vi "GOOP300_GetClassTemplatePath.vi"(1 "ClassTemplateSubDirectory":string, 5 "error in (no error)":errorcluster) -> (15 "FolderPathOut":path, 19 "error out":errorcluster)   [LabVIEW 2016]
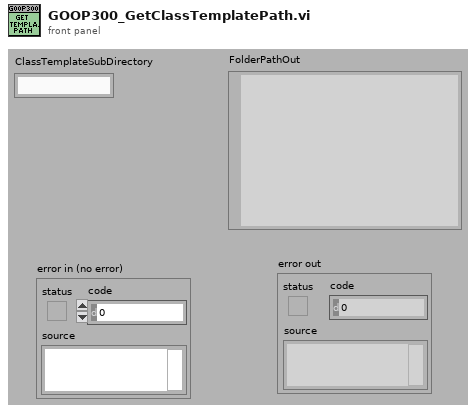
[diagram p1: front panel]
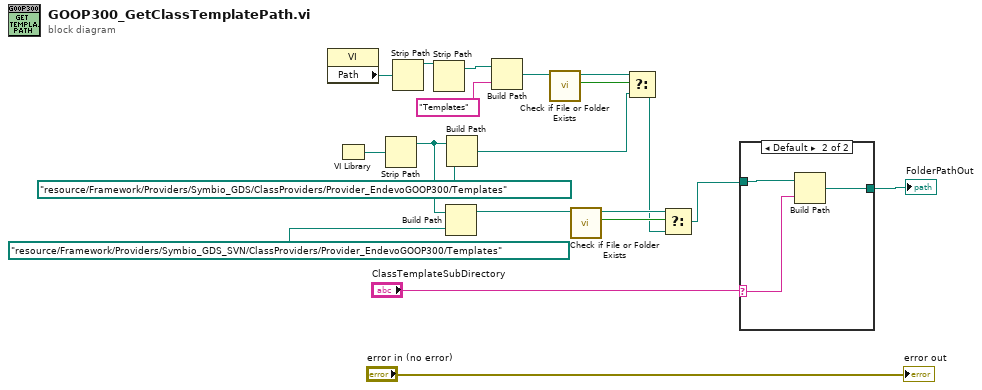
[diagram p0: block diagram]
diagram:
  n1 = property class="VI"() -> ("Path"=w17:path)  [unwired: 2 in, 2 out]
  n2 = VI Library() -> (path=w10:path)
  n3 = Strip Path(path=w10) -> (stripped path=w7:path)  [unwired: 1 out]
  n4 = Strip Path(path=w17) -> (stripped path=w14:path)  [unwired: 1 out]
  n5 = Strip Path(path=w14) -> (stripped path=w20:path)  [unwired: 1 out]
  n6 = Build Path(base path=w7, name or relative path=path "resource/Framework/Providers/Symbio_GDS_SVN/ClassProviders/Provider_EndevoGOOP300/Templates" ("base path")) -> (appended path=w5:path)
  n7 = Build Path(base path=w7, name or relative path=path "resource/Framework/Providers/Symbio_GDS/ClassProviders/Provider_EndevoGOOP300/Templates" ("base path")) -> (appended path=w8:path)
  n8 = Build Path(base path=w20, name or relative path="Templates") -> (appended path=w11:path)
  n9 = call <vilib>:"Check if File or Folder Exists.vi"("path"=w11) -> ("file or folder exists?"=w13:bool, "dup path"=w12:path)  [unwired: 8 in, 1 out]
  n10 = call <vilib>:"Check if File or Folder Exists.vi"("path"=w5) -> ("file or folder exists?"=w4:bool, "dup path"=w3:path)  [unwired: 8 in, 1 out]
  n11 = Select(t=w12, s=w13, f=w8) -> (s? t:f=w2:path)
  n12 = Select(t=w3, s=w4, f=w2) -> (s? t:f=w1:path)
  n13 = case shown="Default" "ClassTemplateSubDirectory" {
    selector: "ClassTemplateSubDirectory" -> [_ w22]
    tunnel: w1 -> [w21 w24]
    tunnel: [w21 w23] -> w19
    frame "" {
    }
    frame Default {
      n14 = Build Path(base path=w24, name or relative path=w22) -> (appended path=w23:path)
    }
  }
  "FolderPathOut" <- w19
  "error out" <- "error in (no error)"
